vi "cdex_Elevation PID.vi"(10 "states":dbl[](array[numeric]) format="%.2f", 11 "elevation":dbl) -> (2 "Output (u)":dbl)   [LabVIEW 2011]
uses:
  <vilib>/Simulation/Implementation/Shared/SIMSCR Execution Mode.ctl
  <vilib>/Simulation/Scripting/Companion Diagram/SimConfigNode/SimParams.ctl
  <vilib>/Simulation/Scripting/Companion Diagram/SimConfigNode/_simSolvers.ctl
  <vilib>/Simulation/Param Hierarchy/Typedefs/SIMPH Param Control Actions.ctl
  <vilib>/Simulation/Implementation/Shared/SIM limit type.ctl
  <vilib>/Simulation/SignalArithmetic/Implementation/NILVSim Gain.llb/SIM Gain (scalar).vi
  <vilib>/Simulation/Nonlinear/Implementation/NILVSim Saturation.llb/SIM Saturation (scalar).vi
  <vilib>/Simulation/ContinuousLinear/Implementation/NILVSim Integrator new.llb/SIM Integrator distributor (scalar).vi
  <vilib>/Simulation/ContinuousLinear/Implementation/NILVSim Integrator new.llb/SIM Integrator collector (scalar).vi
  <vilib>/Simulation/Implementation/Shared/NILVSim_Manager.vi
  <vilib>/Simulation/Implementation/Shared/NILVSim_ParamChanged.vi
  <vilib>/Simulation/Implementation/Shared/NILVSim_FinalizeModel.vi
  <vilib>/Simulation/Implementation/Shared/SIM Unbundle Sim Info.vi
  <vilib>/Simulation/Implementation/Shared/NILVSim_GetModelError.vi
  <vilib>/Simulation/Implementation/Shared/SIM SimErrorHandler.vi
  <vilib>/Simulation/Implementation/Shared/SIM Bundle Sim Info.vi
  3DHe_Global.vi
  <vilib>/Simulation/Implementation/Shared/NILVSim_Initialize.vi
  <vilib>/Simulation/Scripting/Companion Diagram/SimConfigNode/SimDog.xnode
  <vilib>/Simulation/Implementation/XNodeFramework/SimXNode/SimX.xnode
  <vilib>/Simulation/ContinuousLinear/Implementation/NILVSim Integrator new.llb/SIM Integrator (scalar).vi
  <vilib>/Simulation/Implementation/Shared/NI_SIM_Implementation.lvlib
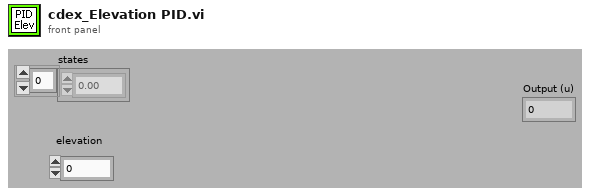
[diagram p1: front panel]
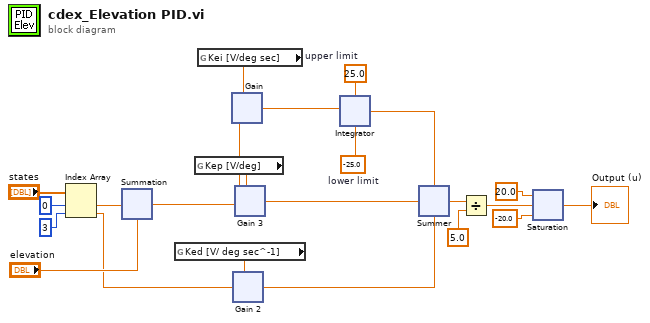
[diagram p0: block diagram]
diagram:
  w11 = -25.0  # lower limit
  w12 = 25.0  # upper limit
  n1 = Index Array(array="states", index #1=0 ("index"), index #2=3 ("index")) -> (element #1=w16:dbl, element #2=w13:dbl)
  n2 = xnode ("Summation")("Operand1"=w16, "Operand2"="elevation") -> ("Result"=w1:dbl)
  n3 = global read "3DHe_Global.vi" "Ked [V/ deg sec^-1]"() -> (w4:dbl)
  n4 = global read "3DHe_Global.vi 3" "Kep [V/deg]"() -> (w3:dbl)
  n5 = global read "3DHe_Global.vi 2" "Kei [V/deg sec]"() -> (w2:dbl)
  n6 = xnode ("Gain")("gain"=w2, "input"=w1) -> ("output"=w21:dbl)  [unwired: 2 in]
  n7 = xnode ("Gain 2")("gain"=w4, "input"=w13) -> ("output"=w14:dbl)  [unwired: 2 in]
  n8 = xnode ("Gain 3")("gain"=w3, "input"=w1) -> ("output"=w22:dbl)  [unwired: 2 in]
  n9 = xnode ("Integrator")("upper limit"=w12, "input"=w21, "lower limit"=w11) -> ("output"=w20:dbl)  [unwired: 7 in, 2 out]
  n10 = xnode ("Summer")("Operand1"=w20, "Operand2"=w22, "Operand3"=w14) -> ("Result"=w9:dbl)
  n11 = Divide(x=w9, y=5.0) -> (x/y=w8:dbl)
  n12 = xnode ("Saturation")("upper limit"=20.0, "input"=w8, "lower limit"=-20.0) -> ("output"=→"Output (u)":dbl)  [unwired: 2 in]
